vi "Calibration.vi"(8 "Error In":errorcluster) -> (0 "Error Out":errorcluster)   [LabVIEW 2017]
panel:
  in  "Sensor 6":dbl
  in  "Sensor 5":dbl
  in  "Sensor 4":dbl
  in  "Sensor 3":dbl
  in  "Sensor 2":dbl
  in  "Sensor 1":dbl
  out "Sensor 1":dynamicdata(graph)
  out "Sensor 5":dynamicdata(graph)
  out "Sensor 2":dynamicdata(graph)
  out "Sensor 3":dynamicdata(graph)
  out "Sensor 4":dynamicdata(graph)
  out "Sensor 6":dynamicdata(graph)
  in  "Home Button":bool
  # "Set Calibration Coefficients"
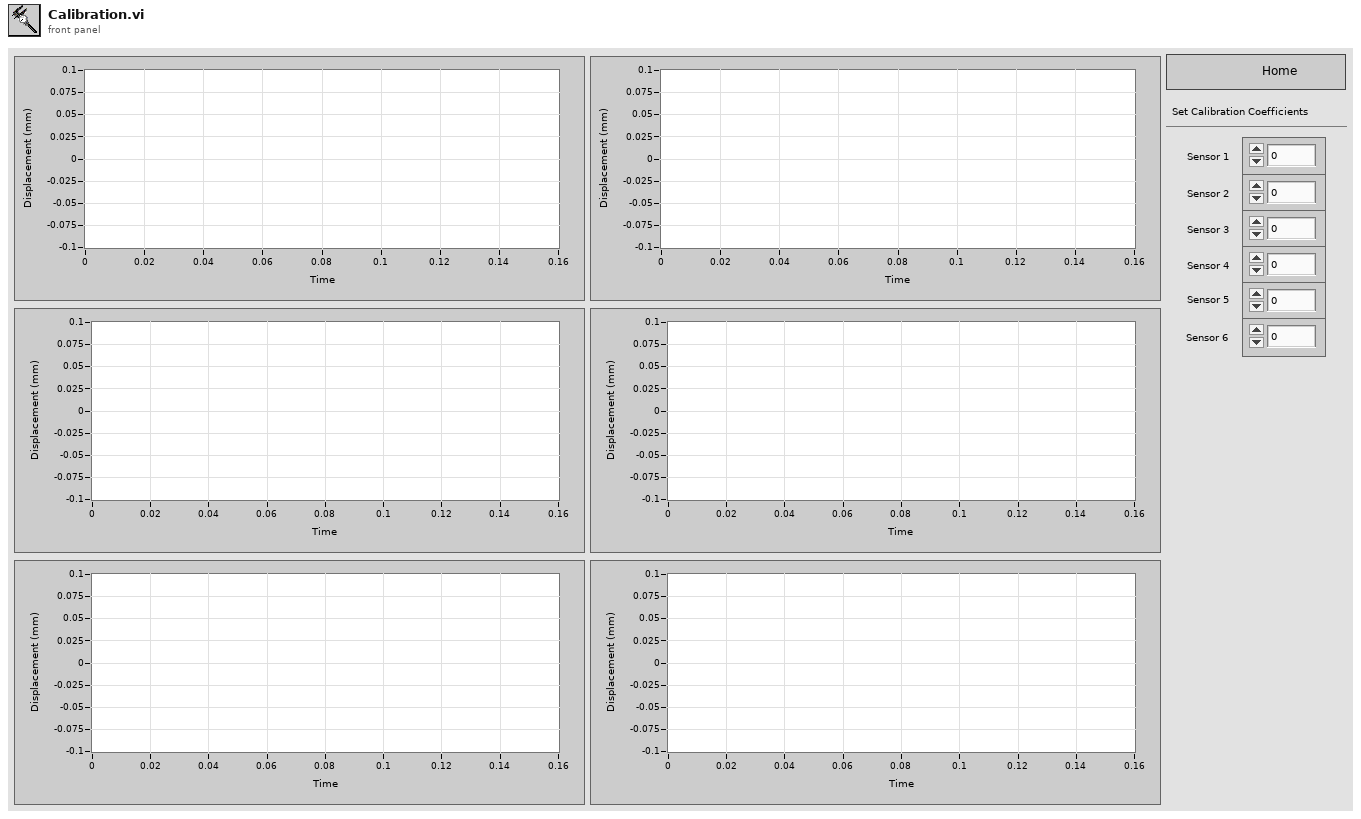
[diagram p1: front panel]
types:
  T1 = enum16{"open", "replace", "create", "open or create", "replace or create", "replace or create with confirmation"}
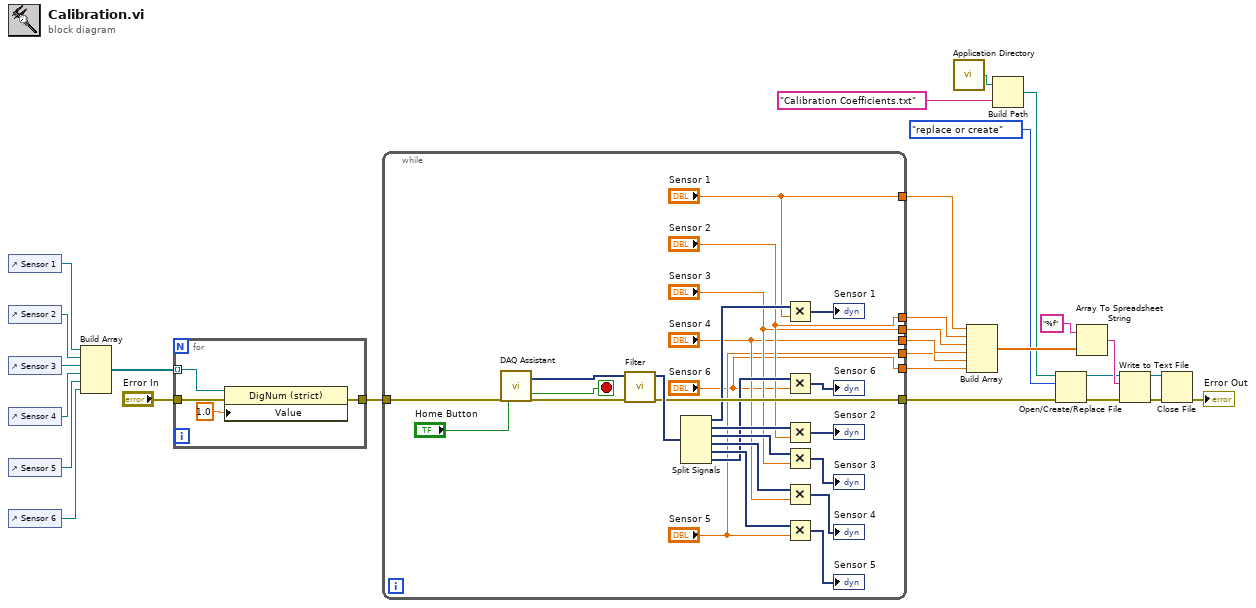
[diagram p0: block diagram]
diagram:
  n1 = control-ref of="Sensor 1"() -> (w9:refnum<vi>)
  n2 = control-ref of="Sensor 2"() -> (w8:refnum<vi>)
  n3 = control-ref of="Sensor 3"() -> (w7:refnum<vi>)
  n4 = control-ref of="Sensor 4"() -> (w6:refnum<vi>)
  n5 = control-ref of="Sensor 5"() -> (w5:refnum<vi>)
  n6 = control-ref of="Sensor 6"() -> (w4:refnum<vi>)
  n7 = Build Array(w9, w8, w7, w6, w5, w4) -> (w3:refnum<vi>[])
  n8 = for {
    tunnel: w3 -> [w32] mode=indexing
    tunnel: [w30] -> w2
    tunnel: "Error In" -> [w29]
    n9 = property class="DigNum (strict)"(reference=w32, error in=w29, "Value"=1.0) -> (error out=w30:errorcluster)  [unwired: 1 out]
  }
  n10 = while {
    tunnel: [w52] -> w14
    tunnel: w2 -> [w51]
    tunnel: ["Sensor 1"] -> w28
    tunnel: ["Sensor 2"] -> w27
    tunnel: ["Sensor 3"] -> w26
    tunnel: ["Sensor 4"] -> w25
    tunnel: ["Sensor 5"] -> w24
    tunnel: ["Sensor 6"] -> w23
    stop <- w55 stop-if-true
    n11 = call "DAQ Assistant"("error in"=w51, "stop (F)"="Home Button") -> ("data"=w57:dynamicdata, "stopped"=w55:bool, "error out"=w54:errorcluster)  [unwired: 14 in, 1 out]
    n12 = call "Filter"("error in (no error)"=w54, "Signal"=w57) -> ("error out"=w52:errorcluster, "Filtered Signal"=w53:dynamicdata)  [unwired: 8 in]
    n13 = Split Signals(w53) -> (w44:dynamicdata, w43:dynamicdata, w42:dynamicdata, w41:dynamicdata, w40:dynamicdata, w39:dynamicdata)  [unwired: 6 in]
    n14 = Multiply(x=w44, y="Sensor 1") -> (x*y=→"Sensor 1":dynamicdata)
    n15 = Multiply(x=w39, y="Sensor 6") -> (x*y=→"Sensor 6":dynamicdata)
    n16 = Multiply(x=w43, y="Sensor 2") -> (x*y=→"Sensor 2":dynamicdata)
    n17 = Multiply(x=w42, y="Sensor 3") -> (x*y=→"Sensor 3":dynamicdata)
    n18 = Multiply(x=w41, y="Sensor 4") -> (x*y=→"Sensor 4":dynamicdata)
    n19 = Multiply(x=w40, y="Sensor 5") -> (x*y=→"Sensor 5":dynamicdata)
  }
  n20 = call <vilib>:"Application Directory.vi"() -> ("Application Directory"=w12:path)
  n21 = Build Array(w28, w27, w26, w25, w24, w23) -> (w22:dbl[])
  n22 = Build Path(base path=w12, name or relative path="Calibration Coefficients.txt") -> (appended path=w10:path)
  n23 = Open/Create/Replace File(file path (use dialog)=w10, error in=w14, operation (0:open)=T1."replace or create") -> (refnum out=w19:refnum<file>, error out=w16:errorcluster)  [unwired: 3 in, 1 out]
  n24 = Array To Spreadsheet String(array=w22, 3:"%f" ("format string")) -> (spreadsheet string=w20:string)  [unwired: 1 in]
  n25 = Write to Text File(file (use dialog)=w19, text=w20, error in=w16) -> (refnum out=w18:refnum<file>, error out=w17:errorcluster)  [unwired: 1 in, 1 out]
  n26 = Close File(refnum=w18, error in=w17) -> (error out=→"Error Out":errorcluster)  [unwired: 1 out]
